vi "Configure RemIO Module.vi"(8 "error in (no error)":errorcluster, 9 "Slave Ref In":refnum<k21>, 10 "11178 in":refnum<class "11178.lvclass">, 11 "Node Ptr In":T1 format="%.0x") -> (0 "error out":errorcluster, 1 "Slave Ref Out":refnum<k21>, 2 "11178 out":refnum<class "11178.lvclass">, 3 "Node Ptr Out":T1 format="%.0x")   [LabVIEW 2016, in "Modules.lvlib" / "11178.lvclass"]
uses:
  11178.lvclass
  <vilib>/NI Veristand/Custom Device API/Custom Device Item Ref.ctl
  11178.lvclass/11178.ctl
  <vilib>/Utility/error.llb/Error Cluster From Error Code.vi
  <vilib>/indcomecat/Remote IO/internal/_Configure REM-11178.vi
  <vilib>/ErrorRing/Error Ring.xnode
  <vilib>/indcomecat/Remote IO/NI ECAT Remote IO.lvlib
  <vilib>/NI Veristand/Custom Device API/Custom Device API.lvlib
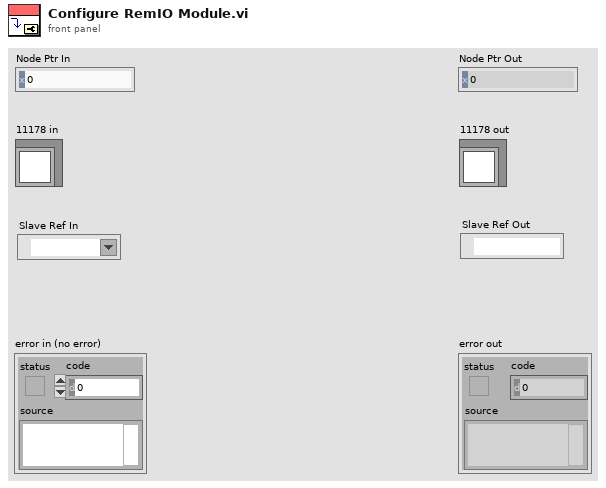
[diagram p1: front panel]
types:
  T1 = typedef "Custom Device API.lvlib/Custom Device Item Ref.ctl" = u64
  T2 = typedef "NI ECAT Remote IO.lvlib/subsititute value on error.ctl" = u8
  T3 = typedef "NI ECAT Remote IO.lvlib/report supply message.ctl" = u8
  T4 = cluster{"substitute value on error":T2, "report \"actuator supply not\npresent\" message?":T3}
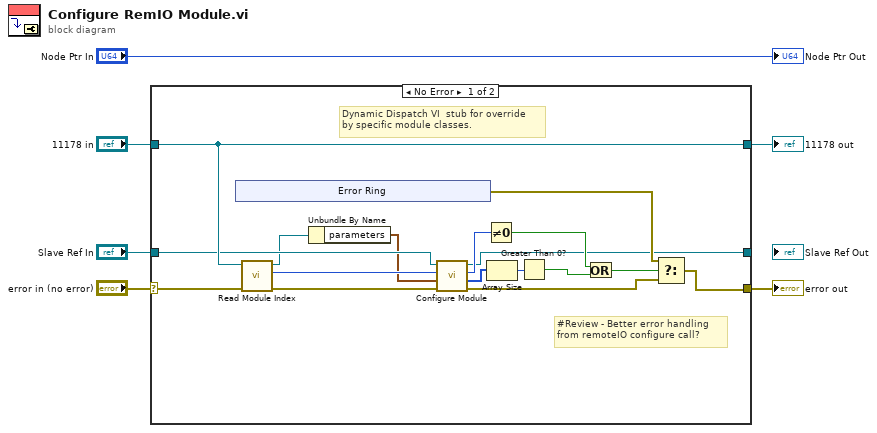
[diagram p0: block diagram]
diagram:
  n1 = case shown="No Error" "error in (no error)" {
    selector: "error in (no error)" -> [w19 w31]
    tunnel: [w20 w31] -> w6
    tunnel: [w17 w30] -> w2
    tunnel: "11178 in" -> [w17 w30]
    tunnel: [w11 w29] -> _
    tunnel: "Slave Ref In" -> [w9 w29]
    frame No Error {
      # "#Review - Better error handling\nfrom remoteIO configure call?"
      # "Dynamic Dispatch VI  stub for override\nby specific module classes."
      n2 = xnode "Error Ring"() -> ("error out"=w21:errorcluster)
      n3 = call-dynamic "Read Module Index.vi"("error in (no error)"=w19, "RemIO Module in"=w17) -> ("error out"=w18:errorcluster, "Module Index"=w10:u8, "RemIO Module out"=w8:refnum<class "11178.lvclass">)  [unwired: 7 in]
      n4 = Unbundle By Name(w8) -> ("parameters"=w7:T4)
      n5 = call-poly <vilib>:"Configure Module.vi"("error in (no error)"=w18, "parameters"=w7, "module slot index"=w10, "slave reference in"=w9) -> ("error out"=w14:errorcluster, "negative confirmation"=w13:u8[], "SDO abort code"=w12:u32, "slave reference out"=w11:refnum<k21>)  [unwired: 4 in]
      n6 = Not Equal To 0?(x=w12) -> (x != 0?=w15:bool)
      n7 = Array Size(array=w13) -> (size(s)=w23:i32)
      n8 = Greater Than 0?(x=w23) -> (x > 0?=w22:bool)
      n9 = Or(x=w15, y=w22) -> (x .or. y?=w16:bool)
      n10 = Select(t=w21, s=w16, f=w14) -> (s? t:f=w20:errorcluster)
    }
    frame Error {
    }
  }
  "error out" <- w6
  "11178 out" <- w2
  "Node Ptr Out" <- "Node Ptr In"
